vi "Multiscale Pyramids.vi"() -> ()   [LabVIEW 2023]
uses:
  <vilib>/vision/NI_Vision_Development_Module.lvlib
  <vilib>/ptbypt/NI_PtbyPt.lvlib
  SubVIs/Parameters Operations.ctl
  SubVIs/ImagesPool Operations TypeDef.ctl
  Images/_Images.ctl
  SubVIs/Conv Flt Presets.ctl
  SubVIs/Unsharp Mask Params TypeDef.ctl
  SubVIs/Multiscale Parameters Typedef.ctl
panel:
  in  "Load":bool
  in  "Save":bool
  in  "MultiScale Parameters":T1={"Preprocessing"=enum."Do Not Process", "Convolution"=enum."Seifert 5x5", "Unsharp Mask Params"={"Amount"=6.0, "Radius"=33.0, "Threshold"=30.0}, "LUT Power"=[0.61538464, 0.43076923, 0.3846154, 0.43846154, 0.42307693, 0.5538462, 0.64615387, 0.61538464, 0.61538464, 0.6, 0.4, 0.4], "LUT Multiplier"=[157.53847, 185.1077, 192.98462, 248.12308, 196.92308, 248.12308, 252.06154, 114.215385, 248.12308, 110.276924, 102.4, 102.4], "Filters"=[enum."Seifert 7x7", enum."Seifert 5x5", enum."Highlight Details 3x3", enum."None", enum."None", enum."None", enum."None", enum."None", enum."None", enum."None", enum."None", enum."None"], "X Value PostProc"=1.2} {"X Value PostProc" scale=0.75..3.0; "LUT Multiplier" scale=0.0..512.0; "LUT Power" scale=0.0..2.0}
  out "mean":dbl format="%0.2f"
  out "Waveform Chart":dbl(graph)
  in  "stop":bool
  out "Time, ms":u32
  out "Pyr Levels":i32=9
  out "Histogram":T4(graph)
  out "Reconstructed\nImage":T5(plugin-control)
  out "Source Image":T5(plugin-control)
  in  "Image":T6=enum."Part1"
  # "Multoscale Contrast Enhancement using Pyramids"
  # "1024x1024"
  # "2048x2048"
  # "4096x4096"
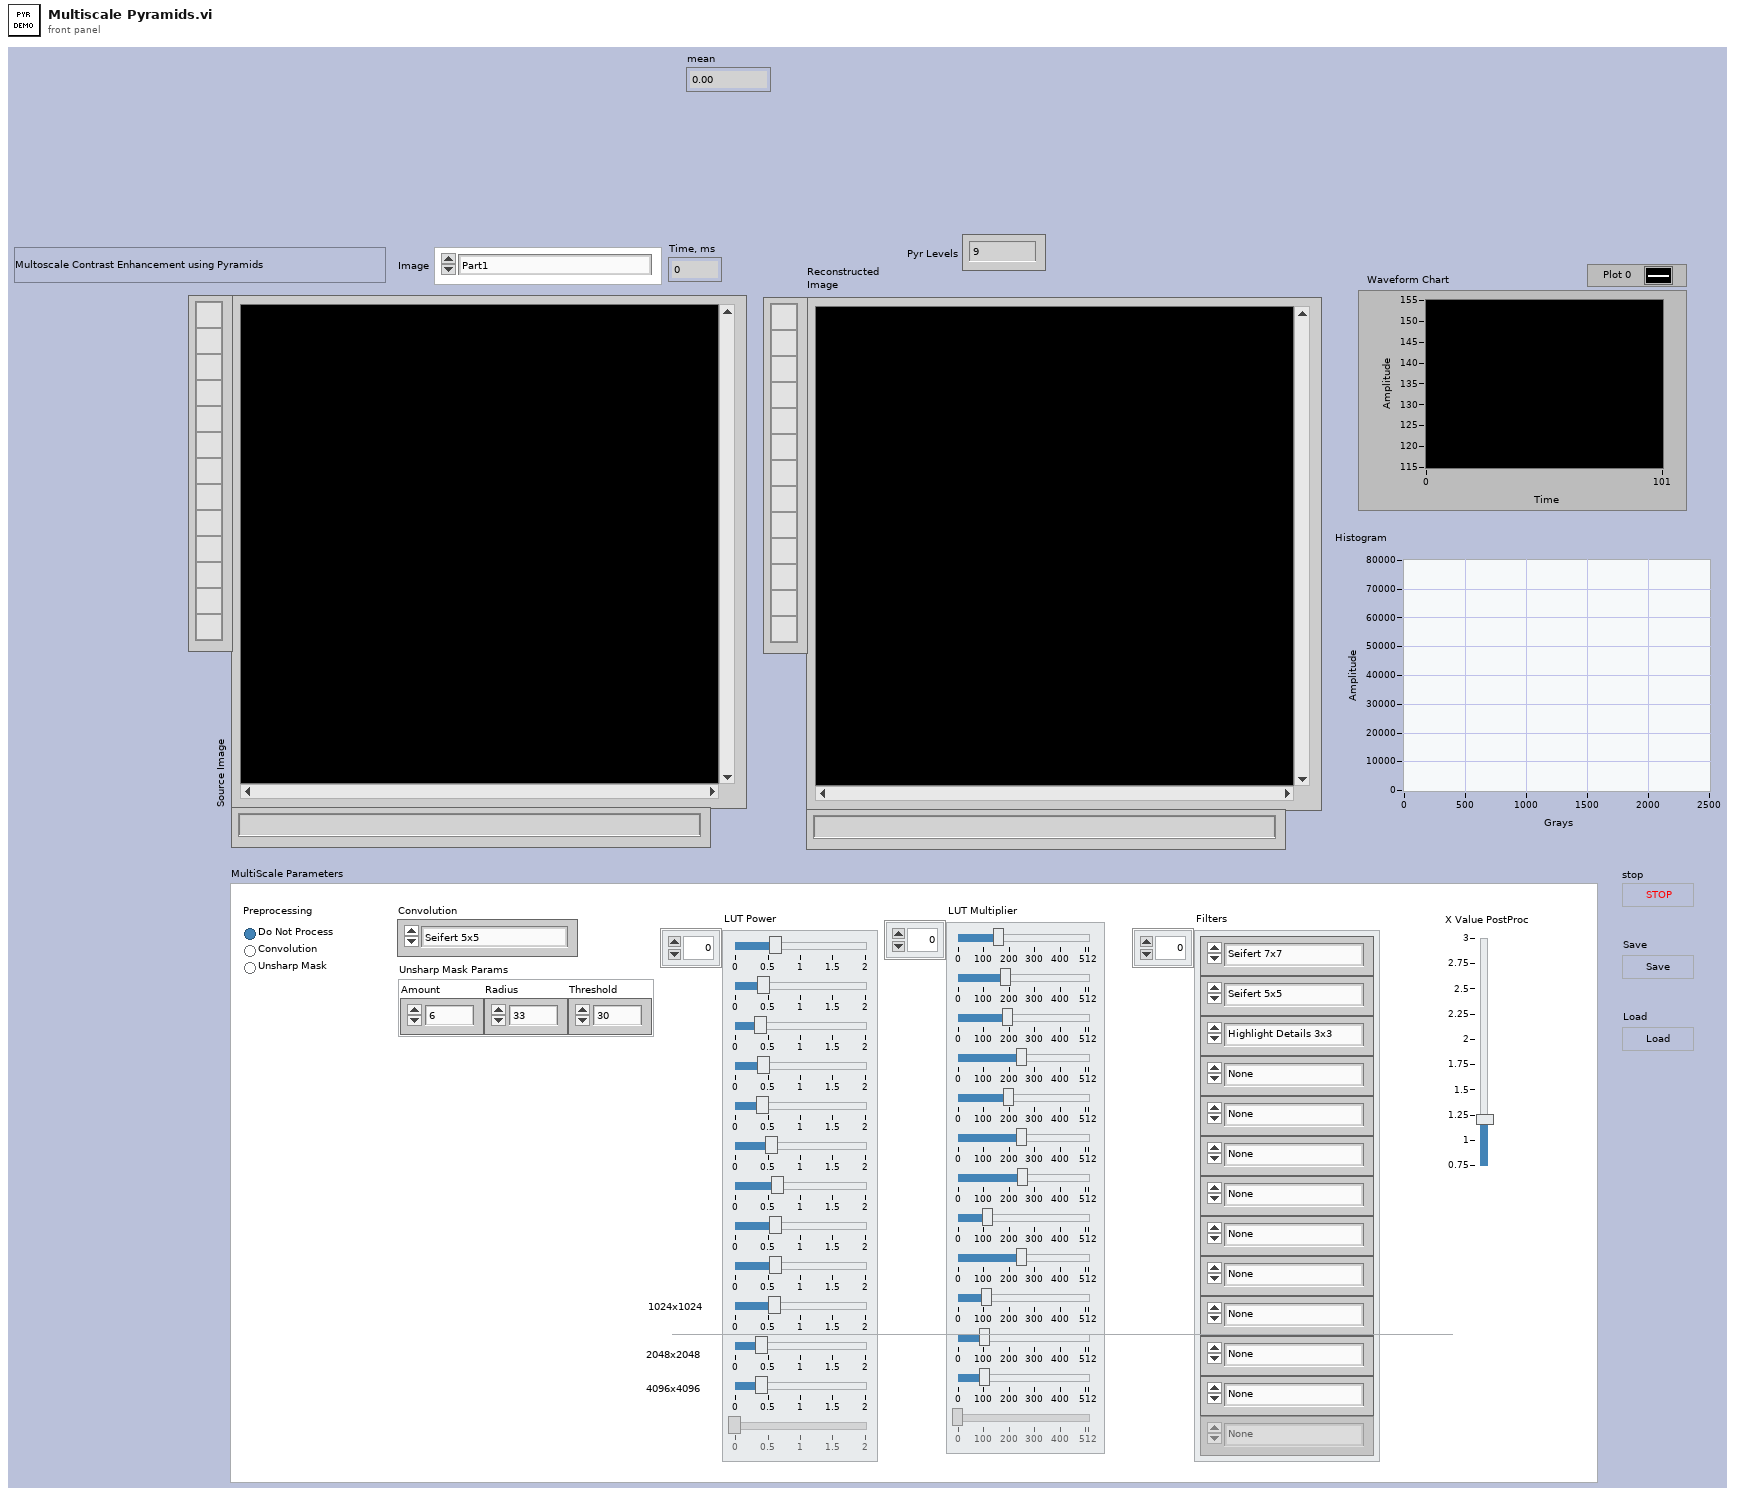
[diagram p1: front panel]
types:
  T1 = typedef "Multiscale Parameters Typedef.ctl" = cluster{"Preprocessing":enum32{"Do Not Process", "Convolution", "Unsharp Mask"}, "Convolution":T2, "Unsharp Mask Params":T3, "LUT Power":sgl[], "LUT Multiplier":sgl[], "Filters":T2[], "X Value PostProc":sgl}
  T2 = typedef "Conv Flt Presets.ctl" = enum16{"None", "Seifert 5x5", "Seifert 7x7", "High Pass 5x5 ", "High Pass 7x7", "Highlight Details 3x3", "Highlight Details 5x5", "Highlight Detail 7x7"}
  T3 = typedef "Unsharp Mask Params TypeDef.ctl" = cluster{"Amount":sgl, "Radius":sgl, "Threshold":sgl}
  T4 = cluster{"Starting Value":sgl, "Incremental Value":sgl, "Histogram":u32[]}
  T5 = typedef "IMAQ Image.ctl" = refnum<image>
  T6 = typedef "_Images.ctl" = enum16{"Ostern2023", "Balls2", "Battery1", "Battery2", "Connector1", "Subwoofer1", "Subwoofer2", "Subwoofer3", "Subwoofer4", "Hase1", "Lamp1", "Lamp2", "Mouse1", "PhotoLens1", "Po1", "PowerSupply1", "Router", "--- Step Wedges ---", "Stepwedge1", "Stepwedge2", "Stepwedge3", "--- PART 01 ---", "Part1", "Part2", "Part3", "Part4", "Part5", "Part6", "Part7", "Part8"}
  T7 = typedef "ImagesPool Operations TypeDef.ctl" = enum16{"Init", "Get Image", "Dispose"}
  T8 = typedef "Image Type" = u32
  T9 = enum32{"Do Not Process", "Convolution", "Unsharp Mask"}
  T10 = typedef "Parameters Operations.ctl" = enum16{"Init", "Get", "Apply", "Save to File", "Load from File"}
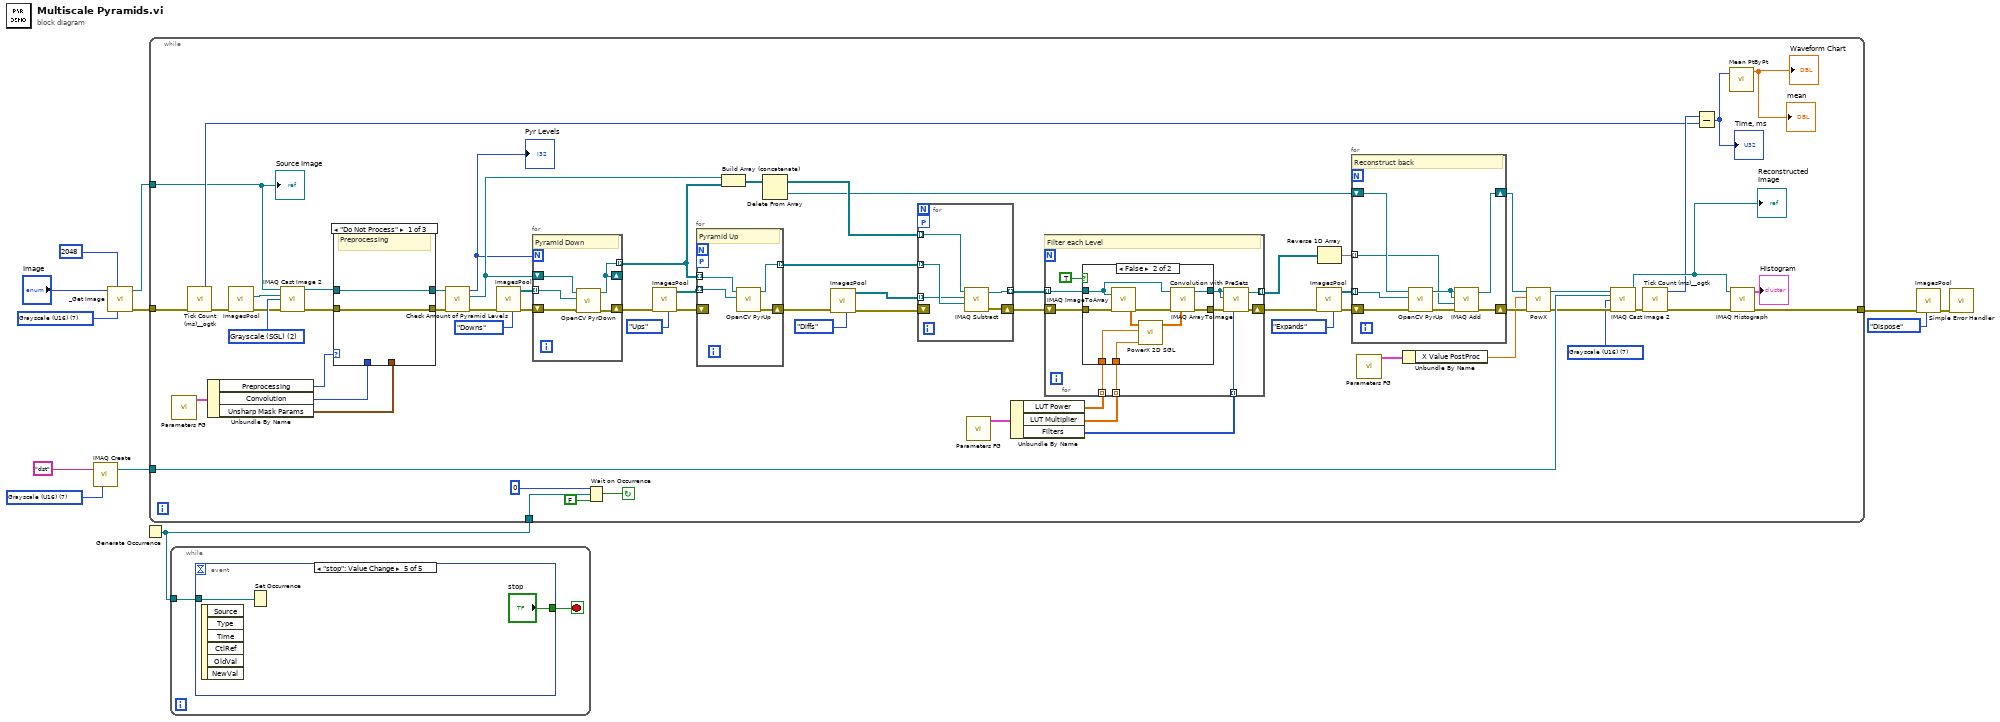
[diagram p0: block diagram]
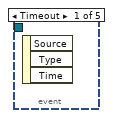
[diagram p2: hidden frame]
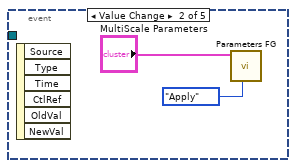
[diagram p3: hidden frame]
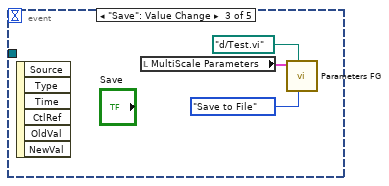
[diagram p4: hidden frame]
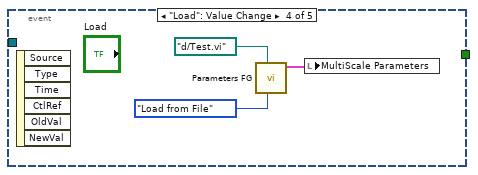
[diagram p5: hidden frame]
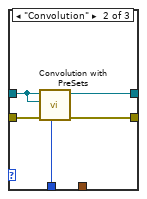
[diagram p6: hidden frame]
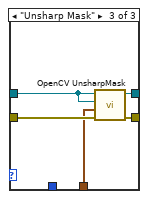
[diagram p7: hidden frame]
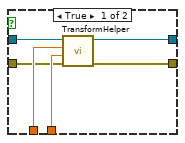
[diagram p8: hidden frame]
diagram:
  w9 = T8 7 items=["Grayscale (U8)", "Grayscale (I16)", "Grayscale (SGL)", "Complex (CSG)", "RGB (U32)", "HSL (U32)", "RGB (U64)", "Grayscale (U16)"] ("Image Type (U16)")
  w11 = T8 7 items=["Grayscale (U8)", "Grayscale (I16)", "Grayscale (SGL)", "Complex (CSG)", "RGB (U32)", "HSL (U32)", "RGB (U64)", "Grayscale (U16)"] ("Image Type")
  n1 = call "IMAQ Create"("Image Name"="dst", "Image Type"=w11) -> ("New Image"=w4:T5)  [unwired: 3 in, 1 out]
  n2 = call "_Get Image.vi"("Image Type (U16)"=w9, "XY Resolution"=2048, "Image"="Image") -> ("error out"=w7:errorcluster, "Image Out"=w6:T5)  [unwired: 5 in, 2 out]
  n3 = Generate Occurrence() -> (w5:refnum<k4>)
  n4 = while {
    tunnel: w4 -> [w60]
    tunnel: w7 -> [w59]
    tunnel: w6 -> [w36]
    tunnel: [w51] -> w2
    tunnel: w5 -> [w40]
    stop <- w39 continue-if-true
    w15 = T8 7 items=["Grayscale (U8)", "Grayscale (I16)", "Grayscale (SGL)", "Complex (CSG)", "RGB (U32)", "HSL (U32)", "RGB (U64)", "Grayscale (U16)"] ("Image Type")
    w38 = T8 2 items=["Grayscale (U8)", "Grayscale (I16)", "Grayscale (SGL)", "Complex (CSG)", "RGB (U32)", "HSL (U32)", "RGB (U64)", "Grayscale (U16)"] ("Image Type")
    n5 = call "Parameters FG.vi"() -> ("MultiScale Parameters Out"=w50:T1)  [unwired: 10 in, 1 out]
    n6 = call <userlib>:"Tick Count (ms)__ogtk.vi"("error in (no error)"=w59) -> ("error out"=w21:errorcluster, "millisecond timer value"=w61:u32)  [unwired: 9 in]
    n7 = Unbundle By Name(w50) -> ("Preprocessing"=w49:T9, "Convolution"=w48:T2, "Unsharp Mask Params"=w47:T3)
    n8 = call "ImagesPool.vi"("error in (no error)"=w21) -> ("error out"=w22:errorcluster, "Filtered Copy"=w37:T5)  [unwired: 8 in, 1 out]
    n9 = call "IMAQ Cast Image 2"("Image Src"=w36, "Image Dst"=w37, "Image Type"=w38, "error in (no error)"=w22) -> ("Image Dst Out"=w34:T5, "error out"=w35:errorcluster)  [unwired: 10 in]
    n10 = case shown="\"Do Not Process\"" w49 {
      tunnel: w34 -> [w80 w82 w86]
      tunnel: [w79 w85 w90] -> w66
      tunnel: [w80 w84 w89] -> w65
      tunnel: w35 -> [w79 w81 w88]
      tunnel: w48 -> [_ w83 _]
      tunnel: w47 -> [_ _ w87]
      frame "Do Not Process" {
        # "Preprocessing"
      }
      frame "Convolution" {
        n11 = call "Convolution with PreSets.vi"("Filter"=w83, "error in (no error)"=w81, "Image Dst"=w82, "Image Src"=w82) -> ("error out"=w85:errorcluster, "Image Dst Out"=w84:T5)  [unwired: 5 in, 1 out]
      }
      frame "Unsharp Mask" {
        n12 = call "OpenCV UnsharpMask.vi"("error in (no error)"=w88, "Unsharp Mask Params"=w87, "Image Dst"=w86, "Image Src"=w86) -> ("error out"=w90:errorcluster, "Image Dst Out"=w89:T5)  [unwired: 5 in, 1 out]
      }
    }
    n13 = call "Check Amount of Pyramid Levels.vi"("error in (no error)"=w66, "Refnum in"=w65) -> ("error out"=w31:errorcluster, "Image Dup"=w64:T5, "Pyr Levels"=w16:i32)  [unwired: 7 in]
    "Pyr Levels" <- w16
    n14 = call "ImagesPool.vi"("Image"=enum16{"Ups", "Downs", "Diffs", "Expands"}."Downs", "error in (no error)"=w31) -> ("error out"=w30:errorcluster, "Array of Images"=w56:T5[])  [unwired: 7 in, 1 out]
    n15 = for {
      N: w16 -> [_]
      shift-right: [w136] -> _
      shift-left: w64 -> [w137]
      tunnel: [w136] -> w69 mode=indexing
      shift-right: [w135] -> w33
      shift-left: w30 -> [w133]
      tunnel: w56 -> [w134] mode=indexing
      # "Pyramid Down"
      n16 = call "OpenCV PyrDown.vi"("error in (no error)"=w133, "Image Dst"=w134, "Image Src"=w137) -> ("error out"=w135:errorcluster, "Image Dst Out"=w136:T5)  [unwired: 7 in]
    }
    n17 = Wait on Occurrence(1:FALSE ("ignore previous (T)"), 2:w40, 3:0 ("ms timeout (-1)")) -> (0:w39:bool)
    n18 = call "ImagesPool.vi"("Image"=enum16{"Ups", "Downs", "Diffs", "Expands"}."Ups", "error in (no error)"=w33) -> ("error out"=w32:errorcluster, "Array of Images"=w55:T5[])  [unwired: 7 in, 1 out]
    n19 = for {
      tunnel: [w132] -> w75 mode=indexing
      tunnel: w69 -> [w131] mode=indexing
      shift-right: [w130] -> w29
      shift-left: w32 -> [_]
      workers-P: _ -> [_]
      tunnel: w55 -> [w129] mode=indexing
      # "Pyramid Up"
      n20 = call "OpenCV PyrUp.vi"("Image Dst"=w129, "Image Src"=w131) -> ("error out"=w130:errorcluster, "Image Dst Out"=w132:T5)  [unwired: 8 in]
    }
    n21 = Build Array (concatenate)(w64, w69) -> (w77:T5[])
    n22 = Delete From Array(array=w77) -> (deleted portion=w74:T5, array with subset deleted=w76:T5[])  [unwired: 2 in]
    n23 = call "ImagesPool.vi"("Image"=enum16{"Ups", "Downs", "Diffs", "Expands"}."Diffs", "error in (no error)"=w29) -> ("error out"=w28:errorcluster, "Array of Images"=w54:T5[])  [unwired: 7 in, 1 out]
    n24 = for {
      tunnel: w76 -> [w128] mode=indexing
      tunnel: w75 -> [w127] mode=indexing
      tunnel: [w126] -> w71 mode=indexing
      shift-right: [w125] -> w68
      shift-left: w28 -> [_]
      workers-P: _ -> [_]
      tunnel: w54 -> [w124] mode=indexing
      n25 = call "IMAQ Subtract"("Image Src A"=w128, "Image Dst"=w124, "Image Src B"=w127) -> ("Image Dst Out"=w126:T5, "error out"=w125:errorcluster)  [unwired: 4 in]
    }
    n26 = call "Parameters FG.vi"() -> ("MultiScale Parameters Out"=w46:T1)  [unwired: 10 in, 1 out]
    n27 = Unbundle By Name(w46) -> ("LUT Power"=w45:sgl[], "LUT Multiplier"=w44:sgl[], "Filters"=w43:T2[])
    n28 = for {
      tunnel: w71 -> [w100] mode=indexing
      tunnel: [w99] -> w72 mode=indexing
      tunnel: w45 -> [w97] mode=indexing
      tunnel: w44 -> [w96] mode=indexing
      shift-right: [w93] -> w27
      shift-left: w68 -> [w94]
      tunnel: w43 -> [w92] mode=indexing
      # "Filter each Level"
      n29 = case shown="False" TRUE {
        tunnel: w100 -> [w106 w115]
        tunnel: [w102 w114] -> w98
        tunnel: w97 -> [w105 w111]
        tunnel: w96 -> [w104 w110]
        tunnel: [w101 w108] -> w95
        tunnel: w94 -> [w103 w107]
        frame True {
          n30 = call "TransformHelper.vi"("error in (no error)"=w103, "Multiplier"=w104, "Power"=w105, "Refnum in"=w106) -> ("error out"=w101:errorcluster, "Refnum out"=w102:T5)  [unwired: 5 in, 1 out]
        }
        frame False {
          n31 = call "IMAQ ImageToArray"("error in (no error)"=w107, "Image"=w115) -> ("Image Pixels (Float)"=w113:sgl[][], "error out"=w109:errorcluster)  [unwired: 2 in, 3 out]
          n32 = call "PowerX 2D SGL.vi"("Multiplier"=w110, "Power"=w111, "Signal In"=w113) -> ("Signal Out"=w112:sgl[][])  [unwired: 8 in]
          n33 = call "IMAQ ArrayToImage"("Image Pixels (Float)"=w112, "error in (no error)"=w109, "Image"=w115) -> ("error out"=w108:errorcluster, "Image Out"=w114:T5)  [unwired: 7 in]
        }
      }
      n34 = call "Convolution with PreSets.vi"("Filter"=w92, "error in (no error)"=w95, "Image Dst"=w98, "Image Src"=w98) -> ("error out"=w93:errorcluster, "Image Dst Out"=w99:T5)  [unwired: 5 in, 1 out]
    }
    n35 = call "ImagesPool.vi"("Image"=enum16{"Ups", "Downs", "Diffs", "Expands"}."Expands", "error in (no error)"=w27) -> ("error out"=w26:errorcluster, "Array of Images"=w53:T5[])  [unwired: 7 in, 1 out]
    n36 = Reverse 1D Array(array=w72) -> (reversed array=w73:T5[])
    n37 = for {
      shift-right: [w120] -> w70
      shift-left: w74 -> [w123]
      tunnel: w73 -> [w121] mode=indexing
      shift-right: [w117] -> w67
      shift-left: w26 -> [w119]
      tunnel: w53 -> [w116] mode=indexing
      # "Reconstruct back"
      n38 = call "OpenCV PyrUp.vi"("error in (no error)"=w119, "Image Dst"=w116, "Image Src"=w123) -> ("error out"=w118:errorcluster, "Image Dst Out"=w122:T5)  [unwired: 7 in]
      n39 = call "IMAQ Add"("Image Src A"=w122, "Image Dst"=w122, "Image Src B"=w121, "error in (no error)"=w118) -> ("Image Dst Out"=w120:T5, "error out"=w117:errorcluster)  [unwired: 3 in]
    }
    n40 = call "Parameters FG.vi"() -> ("MultiScale Parameters Out"=w42:T1)  [unwired: 10 in, 1 out]
    n41 = Unbundle By Name(w42) -> ("X Value PostProc"=w41:sgl)
    n42 = call "PowX.vi"("error in (no error)"=w67, "X Value"=w41, "Refnum in"=w70) -> ("error out"=w25:errorcluster, "Refnum out"=w63:T5)  [unwired: 7 in]
    n43 = call "IMAQ Cast Image 2"("Image Src"=w63, "Image Dst"=w60, "Image Type"=w15, "error in (no error)"=w25) -> ("Image Dst Out"=w78:T5, "error out"=w24:errorcluster)  [unwired: 10 in]
    "Reconstructed\nImage" <- w78
    n44 = call <userlib>:"Tick Count (ms)__ogtk.vi"("error in (no error)"=w24) -> ("error out"=w23:errorcluster, "millisecond timer value"=w62:u32)  [unwired: 9 in]
    n45 = Subtract(x=w62, y=w61) -> (x-y=w58:u32)
    "Time, ms" <- w58
    n46 = call <vilib>:"Mean PtByPt.vi"("x"=w58) -> ("mean"=→"Waveform Chart" →"mean":dbl)  [unwired: 3 in, 1 out]
    n47 = call "IMAQ Histograph"("error in (no error)"=w23, "Image"=w78) -> ("error out"=w51:errorcluster, "Histogram Graph"=→"Histogram":T4)  [unwired: 6 in, 2 out]
    "Source Image" <- w36
  }
  n48 = while {
    tunnel: w5 -> [w138]
    stop <- w139 stop-if-true
    n49 = event shown="[4] \"stop\": Value Change" {
      selector: _ -> [_ _ _ _ _]
      dyn-events: _ -> [_ _ _ _ _]
      timeout: _ -> [_ _ _ _ _]
      tunnel: [_ _ _ _ "stop"] -> w139
      tunnel: w138 -> [_ _ _ _ w148]
      event Timeout {
        n50 = event-data() -> ()  [unwired: 1 in, 3 out]
      }
      event Value Change {
        n51 = event-data() -> ()  [unwired: 1 in, 6 out]
        n52 = call "Parameters FG.vi"("Params Operations (Get)"=Parameters_Operations."Apply" ("Params Operations"), "MultiScale Parameters In"="MultiScale Parameters") -> ()  [unwired: 8 in, 2 out]
      }
      event "Save": Value Change {
        n53 = event-data() -> ()  [unwired: 1 in, 6 out]
        n54 = local read "MultiScale Parameters"() -> (w142:T1)
        n55 = call "Parameters FG.vi"("Params Operations (Get)"=Parameters_Operations."Save to File", "configuration file path"=path "d:/Test.vi", "MultiScale Parameters In"=w142) -> ()  [unwired: 7 in, 2 out]
      }
      event "Load": Value Change {
        n56 = event-data() -> ()  [unwired: 1 in, 6 out]
        n57 = call "Parameters FG.vi"("Params Operations (Get)"=Parameters_Operations."Load from File", "configuration file path"=path "d:/Test.vi") -> ("MultiScale Parameters Out"=w145:T1)  [unwired: 8 in, 1 out]
        n58 = local write "MultiScale Parameters"(w145) -> ()
      }
      event "stop": Value Change {
        n59 = event-data() -> ()  [unwired: 1 in, 6 out]
        n60 = Set Occurrence(w148) -> ()
      }
    }
  }
  n61 = call "ImagesPool.vi"("Op"=ImagesPool_Operations_TypeDef."Dispose", "error in (no error)"=w2) -> ("error out"=w1:errorcluster)  [unwired: 7 in, 2 out]
  n62 = call <vilib>:"Simple Error Handler.vi"("error in (no error)"=w1) -> ()  [unwired: 4 in, 5 out]
